vi "Actor Core.vi"(8 "error in":errorcluster, 11 "Context in":refnum<class "Context.lvclass">) -> (0 "error out":errorcluster, 3 "Actor out":refnum<class "Actor.lvclass">)   [LabVIEW 2021, in "Context.lvlib" / "Context.lvclass"]
doc: "(<B>Filename</B>: Actor Framework.lvlib:Actor.lvclass:Actor Core.vi)\n\nReceives messages to the actor, reacts to them, and initiates any error handling that may shut the actor down.\n\nDescendant classes may override this VI to append parallel tasks for the actor to complete while it handles messages. Overrides use the Call Parent Method node."
uses:
  Context.lvclass
  C:/PPLs/Design-Patterns/State Pattern/State Pattern/State Pattern/State Pattern.lvclass
  C:/Program Files/National Instruments/LabVIEW 2021/vi.lib/ActorFramework/Actor/Actor.lvclass
  <vilib>/ActorFramework/Actor/Actor.lvclass
  A State/A State.lvclass
  C:/PPLs/Design-Patterns/State Pattern/Example/Context/State/State.lvclass
  Context.lvclass/Context.ctl
  <vilib>/ActorFramework/Actor/Actor.lvclass/Actor.ctl
  <vilib>/ActorFramework/Message Enqueuer/Message Enqueuer.lvclass/Message Enqueuer.ctl
  B State/B State.lvclass
  C:/PPLs/Design-Patterns/State Pattern/State Pattern/State Change Core/State Change Core/State Change Core.lvclass
  State Pattern/State Change Core/State Change Core Messages/State Change Core Msg/State Change Core Msg.lvclass/State Change Core Msg.ctl
  <vilib>/ActorFramework/Message Enqueuer/Init from Existing Queue.vi
  <vilib>/ActorFramework/Message Enqueuer/Enqueue.vi
  <vilib>/ActorFramework/Stop Msg/Stop Msg.lvclass
  C:/Program Files/National Instruments/LabVIEW 2021/vi.lib/ActorFramework/Message/Message.lvclass
  Messages/xxxx/xxxx Messages/xxxx Msg/xxxx Msg.lvclass
  Messages/Flip States/Flip States Messages/Flip States Msg/Flip States Msg.lvclass
  State Pattern/State Change Core/State Change Core Messages/State Change Core Msg/State Change Core Msg.lvclass
  <vilib>/ActorFramework/Message Priority Queue/Priority Enqueue.vi
  <vilib>/ActorFramework/Message Enqueuer/Message Enqueuer.lvclass
  State Pattern/State Pattern/State Pattern.lvclass
panel:
  in  "Change to B Context State":bool
  in  "Flip States":bool
  out "Current Context I32":i32
  out "Current State":string
  in  "Send Self the xxxx Msg":bool
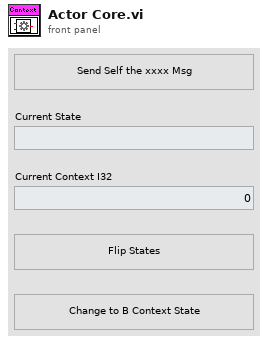
[diagram p1: front panel]
types:
  T1 = cluster{"Stop":refnum<user-event>, "Current State":refnum<user-event>, "Current Context I32":refnum<user-event>}
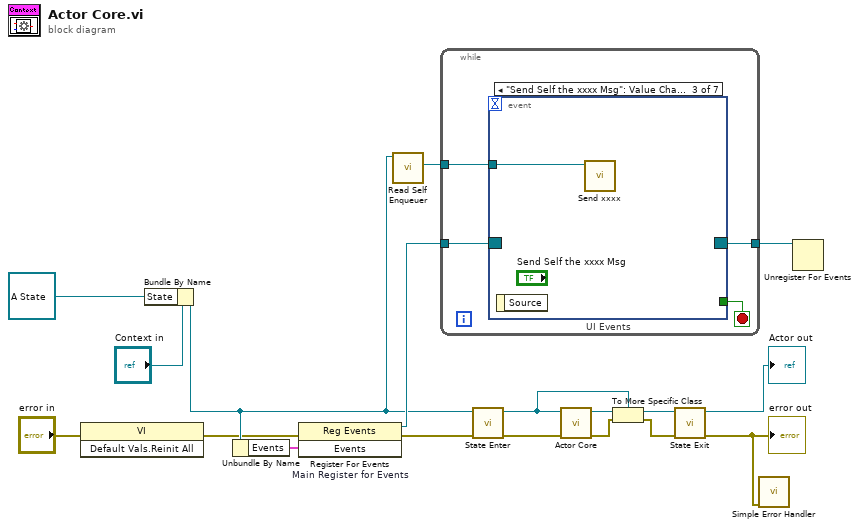
[diagram p0: block diagram]
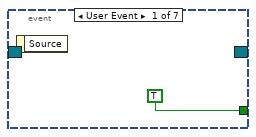
[diagram p2: hidden frame]
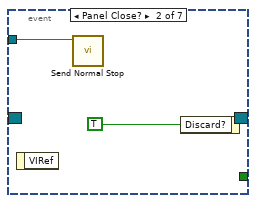
[diagram p3: hidden frame]
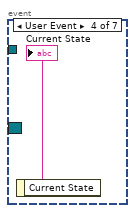
[diagram p4: hidden frame]
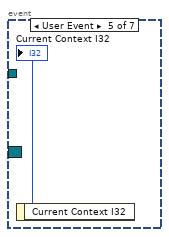
[diagram p5: hidden frame]
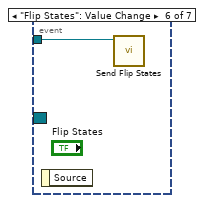
[diagram p6: hidden frame]
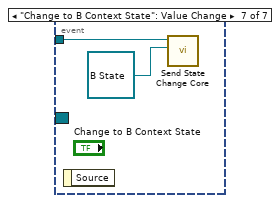
[diagram p7: hidden frame]
diagram:
  n1 = invoke class="VI" method="Default Vals.Reinit All"(error in="error in") -> (error out=w4:errorcluster)  [unwired: 2 in, 2 out]
  n2 = Bundle By Name(cluster="Context in", "State"=refnum<class "A State.lvclass"> refnum ("Context Actor.lvlib:A Context State.lvclass")) -> (w5:refnum<class "Context.lvclass">)
  n3 = Unbundle By Name(w5) -> ("Events"=w18:T1)
  n4 = register-events "Main Register for Events"(error in=w4, w18) -> (reference out=w9:refnum<event-registration>, error out=w8:errorcluster)  [unwired: 1 in]
  n5 = call <vilib>:"Read Self Enqueuer.vi"("Actor"=w5) -> ("Self Enqueuer"=w16:refnum<class "Message Enqueuer.lvclass">)  [unwired: 10 in]
  n6 = while {
    tunnel: w9 -> [w22]
    tunnel: [w20] -> w17
    tunnel: w16 -> [w19]
    stop <- w21 stop-if-true
    n7 = event "UI Events" shown="[2] \"Send Self the xxxx Msg\": Value Change" {
      selector: w22 -> [_ _ _ _ _ _ _]
      dyn-events: [_ _ _ _ _ _ _] -> w20
      timeout: _ -> [_ _ _ _ _ _ _]
      tunnel: [TRUE _ _ _ _ _ _] -> w21
      tunnel: w19 -> [_ w24 w26 _ _ w29 w31]
      event User Event {
        n8 = event-data() -> ()  [unwired: 1 in, 1 out]
      }
      event Panel Close? {
        n9 = event-data() -> ()  [unwired: 1 in, 1 out]
        n10 = call <vilib>:"Send Normal Stop.vi"("Message Enqueuer"=w24) -> ()  [unwired: 10 in, 1 out]
        n11 = event-data("Discard?"=TRUE) -> ()  [unwired: 1 in, 1 out]
      }
      event "Send Self the xxxx Msg": Value Change {
        n12 = event-data() -> ()  [unwired: 1 in, 1 out]
        n13 = call "Send xxxx.vi"("Message Enqueuer"=w26) -> ()  [unwired: 9 in, 2 out]
      }
      event User Event {
        n14 = event-data() -> ("Current State"=→"Current State":string)  [unwired: 1 in]
      }
      event User Event {
        n15 = event-data() -> ("Current Context I32"=→"Current Context I32":i32)  [unwired: 1 in]
      }
      event "Flip States": Value Change {
        n16 = event-data() -> ()  [unwired: 1 in, 1 out]
        n17 = call "Send Flip States.vi"("Message Enqueuer"=w29) -> ()  [unwired: 9 in, 2 out]
      }
      event "Change to B Context State": Value Change {
        n18 = event-data() -> ()  [unwired: 1 in, 1 out]
        n19 = call "Send State Change Core.vi"("Transition State"=refnum<class "B State.lvclass"> refnum ("Context.lvlib:B Context State.lvclass"), "Message Enqueuer"=w31) -> ()  [unwired: 8 in, 2 out]
      }
    }
  }
  n20 = call "State Enter.vi"("error in"=w8, "State in"=w5) -> ("error out"=w7:errorcluster, "State out"=w6:refnum<class "Context.lvclass">)  [unwired: 8 in]
  n21 = call-parent "Actor Core.vi"("error in"=w7, "Actor in"=w6) -> ("error out"=w2:errorcluster, "Actor out"=w15:refnum<class "Actor.lvclass">)  [unwired: 8 in]
  n22 = To More Specific Class(target class=w6, reference=w15, error in=w2) -> (specific class reference=w11:refnum<class "Context.lvclass">, error out=w1:errorcluster)
  n23 = call "State Exit.vi"("error in"=w1, "State in"=w11) -> ("error out"=w10:errorcluster, "State out"=→"Actor out":refnum<class "Context.lvclass">)  [unwired: 8 in]
  "error out" <- w10
  n24 = call <vilib>:"Simple Error Handler.vi"("error in (no error)"=w10) -> ()  [unwired: 4 in, 5 out]
  n25 = Unregister For Events(event registration refnum=w17) -> ()  [unwired: 1 in, 1 out]
